vi "DSB Modulation Demo (Baseband-Sine) - BasicMozart.vi"() -> ()   [LabVIEW 2013]
uses:
  <vilib>/sound2/lvsound2.llb/Sound File Info (path).vi
  <vilib>/sound2/lvsound2.llb/Sound File Read Open.vi
  <vilib>/sound2/lvsound2.llb/Sound File Read (DBL).vi
  <vilib>/Waveform/WDTOps.llb/WDT Get Waveform Subset DBL.vi
  <vilib>/express/express analysis/Spectral/Block/exnSpectralBlock spectral measurements power poly.vi
  <vilib>/express/express analysis/Spectral/Block/exnSpectralBlock spectral measurements power DDT.vi
  <vilib>/express/express analysis/Spectral/XNode/ExpressSpectralMeasurementsBlockNode.xnode
panel:
  in  "Path":path=path "D:/wendy/study/2023-2024Spring/EE206lab/lab2/mozart.wav"
  in  "Duration":dbl=44101.0 caption="Frequency"
  in  "Resample Rate":dbl=1000000.0 caption="Frequency"
  in  "WAV Sample Rate":dbl=44100.0 caption="dt"
  in  "LPF Cut-Off":dbl=10000.0 caption="Lower Cut-Off"
  in  "SNR (dB)":dbl(slide)=30.0 caption="Standard deviation" scale=-20.0..30.0
  out "Comparision":dynamicdata(graph)
  out "Baseband":dynamicdata(graph)
  out "DSB FFT":dynamicdata(graph)
  out "DSB Wave":dynamicdata(graph)
  in  "Carrier Amp.":dbl=1.0 caption="Amplitude"
  in  "stop":bool
  in  "Frequency Offset":dbl(slide) scale=0.0..1000.0
  in  "Carrier Freq.":dbl=100000.0 caption="Frequency"
  # "DSB Modulation"
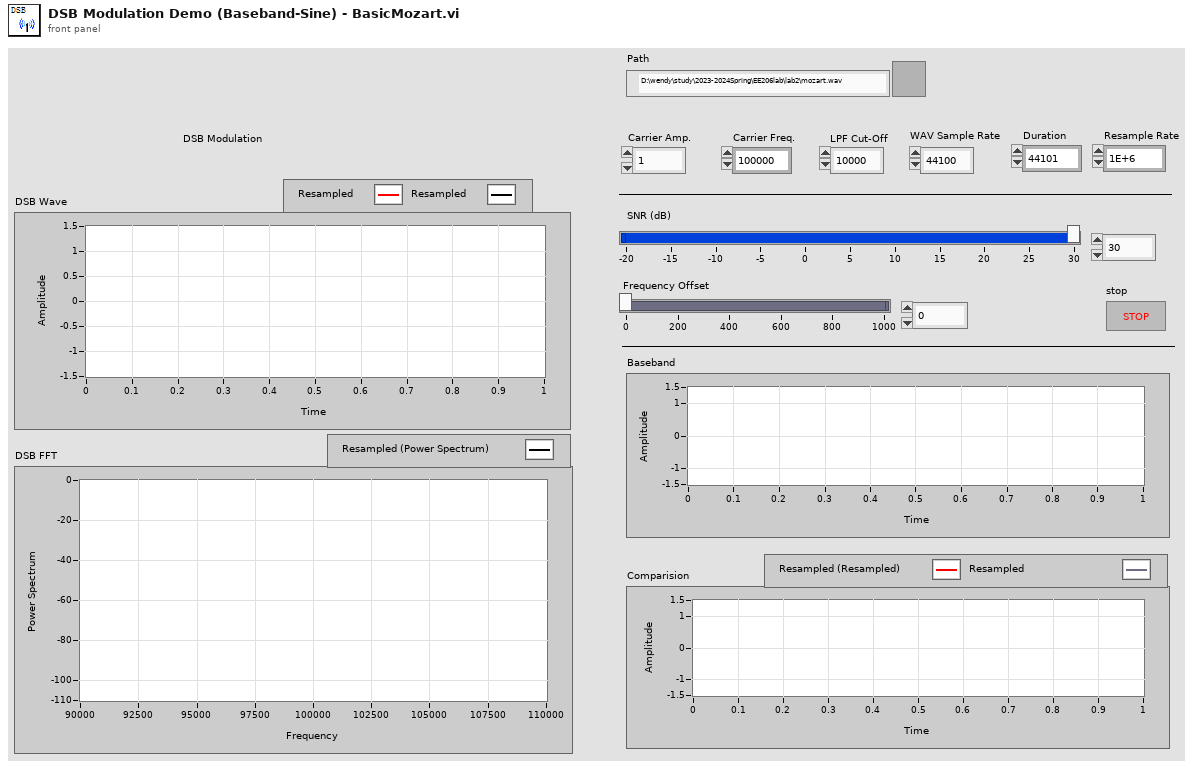
[diagram p1: front panel]
types:
  T1 = typedef "Sound File Refnum.ctl" = refnum<file>
  T2 = cluster{"averaging mode":u16, "weighting mode":u16, "number of averages":u32}
  T3 = cluster{"dB On (F)":bool, "unwrap phase (F)":bool, "convert to degree (F)":bool}
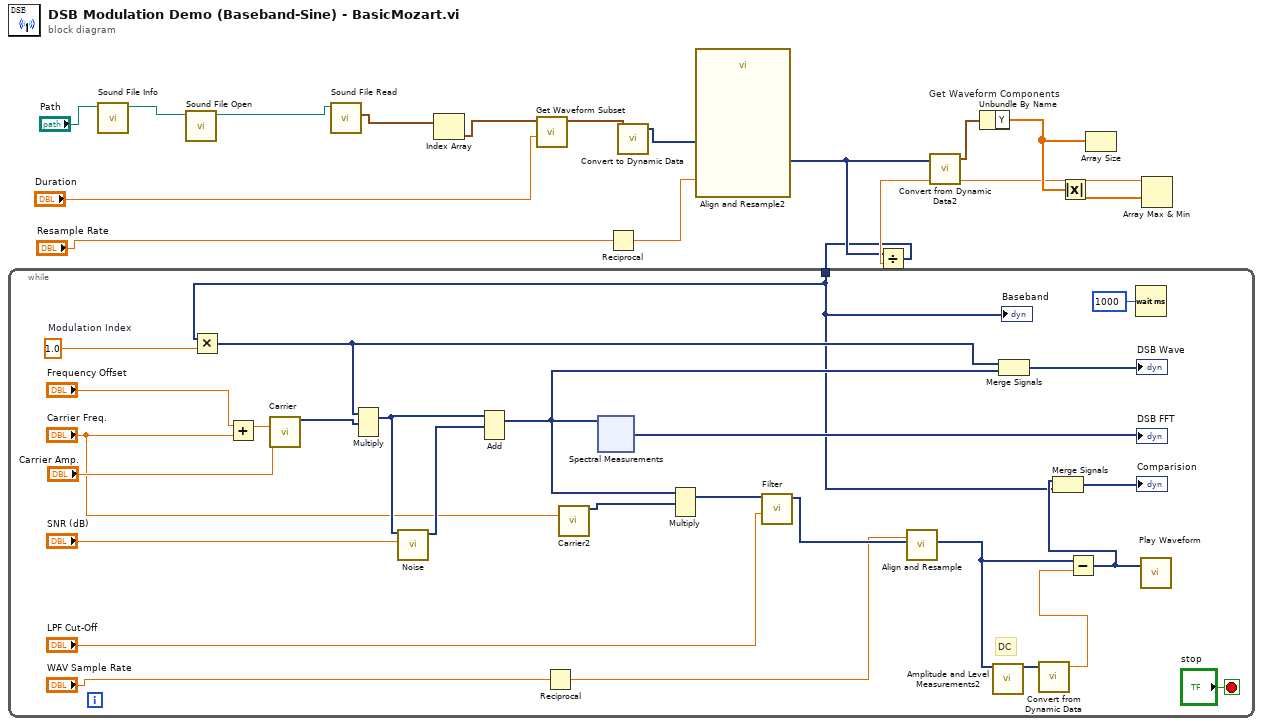
[diagram p0: block diagram]
diagram:
  n1 = call-poly <vilib>:"Sound File Info.vi"("path"="Path") -> ("path out"=w6:path)  [unwired: 7 in, 3 out]
  n2 = call-poly <vilib>:"Sound File Open.vi"("path"=w6) -> ("sound file refnum"=w15:T1)  [unwired: 9 in, 1 out]
  n3 = call-poly <vilib>:"Sound File Read.vi"("sound file refnum"=w15) -> ("data"=w14:waveform(dbl)[])  [unwired: 6 in, 4 out]
  n4 = Index Array "Index Array"(array=w14) -> (element=w13:waveform(dbl))  [unwired: 1 in]
  n5 = call-poly <vilib>:"Get Waveform Subset.vi"("duration"="Duration", "waveform in"=w13) -> ("waveform out"=w7:waveform(dbl))  [unwired: 4 in, 3 out]
  n6 = Reciprocal(x="Resample Rate") -> (1/x=w8:dbl)
  n7 = call "Convert to Dynamic Data"("Waveform"=w7) -> ("Dynamic Data Type"=w12:dynamicdata)  [unwired: 3 in]
  n8 = call "Align and Resample2"("dt"=w8, "Signals"=w12) -> ("Resampled Signals"=w5:dynamicdata)  [unwired: 7 in, 2 out]
  n9 = call "Convert from Dynamic Data2"("Dynamic Data Type"=w5) -> ("Waveform"=w4:waveform(dbl))  [unwired: 3 in]
  n10 = Unbundle By Name "Get Waveform Components"(w4) -> ("Y"=w11:dbl[])
  n11 = Absolute Value(x=w11) -> (abs(x)=w10:dbl[])
  n12 = Array Size(array=w11) -> ()  [unwired: 1 out]
  n13 = Array Max & Min(array=w10) -> (max value=w9:dbl)  [unwired: 3 out]
  n14 = Divide(x=w5, y=w9) -> (x/y=w1:dynamicdata)
  n15 = while {
    tunnel: w1 -> [w17]
    stop <- "stop" stop-if-true
    w37 = 1.0  # Modulation Index
    # "DC"
    n16 = Multiply(x=w17, y=w37) -> (x*y=w33:dynamicdata)
    n17 = Add(x="Frequency Offset", y="Carrier Freq.") -> (x+y=w36:dbl)
    n18 = call "Carrier"("Frequency"=w36, "Amplitude"="Carrier Amp.") -> ("Sine"=w34:dynamicdata)  [unwired: 12 in, 1 out]
    n19 = Multiply(1:w34, 2:w33) -> (0:w31:dynamicdata)  [unwired: 1 in, 1 out]
    n20 = call "Noise.vi"("AWGN (dB)"="SNR (dB)", "Dynamic Data"=w31) -> ("DC with Gaussian Noise"=w32:dynamicdata)  [unwired: 9 in]
    n21 = Add(1:w32, 2:w31) -> (0:w26:dynamicdata)  [unwired: 1 in, 1 out]
    n22 = Reciprocal(x="WAV Sample Rate") -> (1/x=w18:dbl)
    n23 = call "Carrier2"("Frequency"="Carrier Freq.") -> ("Sine"=w27:dynamicdata)  [unwired: 13 in, 1 out]
    n24 = xnode "Spectral Measurements"("Signals"=w26) -> ("Power Spectrum"=→"DSB FFT":dynamicdata)  [unwired: 2 in, 2 out]
    n25 = Multiply(1:w27, 2:w26) -> (0:w25:dynamicdata)  [unwired: 1 in, 1 out]
    n26 = call "Filter"("Lower Cut-Off"="LPF Cut-Off", "Signal"=w25) -> ("Filtered Signal"=w24:dynamicdata)  [unwired: 8 in, 1 out]
    n27 = call "Align and Resample"("dt"=w18, "Signals"=w24) -> ("Resampled Signals"=w40:dynamicdata)  [unwired: 7 in, 2 out]
    n28 = call "Amplitude and Level Measurements2"("Signals"=w40) -> ("Mean (DC)"=w42:dynamicdata)  [unwired: 13 in, 1 out]
    n29 = Merge Signals(w33, w26) -> (→"DSB Wave":dynamicdata)
    n30 = call "Convert from Dynamic Data"("Dynamic Data Type"=w42) -> ("Scalar"=w39:dbl)  [unwired: 3 in]
    n31 = Subtract(x=w40, y=w39) -> (x-y=w22:dynamicdata)
    n32 = Merge Signals(w22, w17) -> (→"Comparision":dynamicdata)
    n33 = Wait (ms)(milliseconds to wait=u32 1000) -> ()  [unwired: 1 out]
    n34 = call "Play Waveform"("Data"=w22) -> ()  [unwired: 18 in, 1 out]
    "Baseband" <- w17
  }
